vi "Heat Flow Front Panel.vi"(3 "Temp Control":dbl) -> (11 "Temp Indicator":dbl)   [LabVIEW 2019, in "Test Stands.lvlib" / "Heat Flow Test Stand.lvclass"]
uses:
  Heat Flow Test Stand.lvclass
panel:
  out "Heater dU":dbl format="%#.3f"
  out "Hot Side I":dbl format="%#.3f"
  out "I Res dU":dbl format="%#.1f"
  in  "ColdSideVolts":dbl min=0.0 max=8.0 step=0.01
  in  "HotSideVolts":dbl min=0.0 max=8.0 step=0.01
  out "Hot Side Power":dbl format="%9.2f"
  out "Hot Side Temp":dbl format="%#.2f"
  out "Cold Side Temp":dbl format="%#.2f"
  out "T 1":dbl
  out "T 2":dbl
  out "T 3":dbl
  out "T 4":dbl
  out "T 5":dbl
  out "T 6":dbl
  out "T 7":dbl
  out "T 8":dbl
  # "K"
  # "mV"
  # "A"
  # "V"
  # "K"
  # "W"
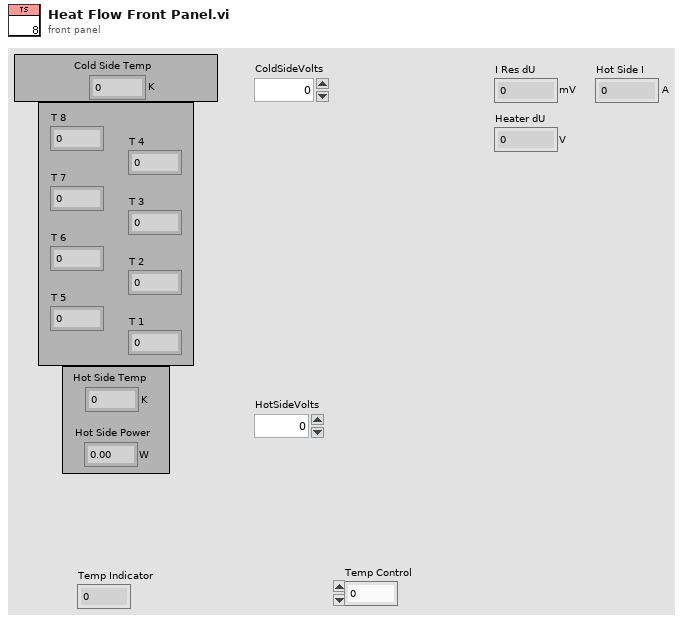
[diagram p1: front panel]
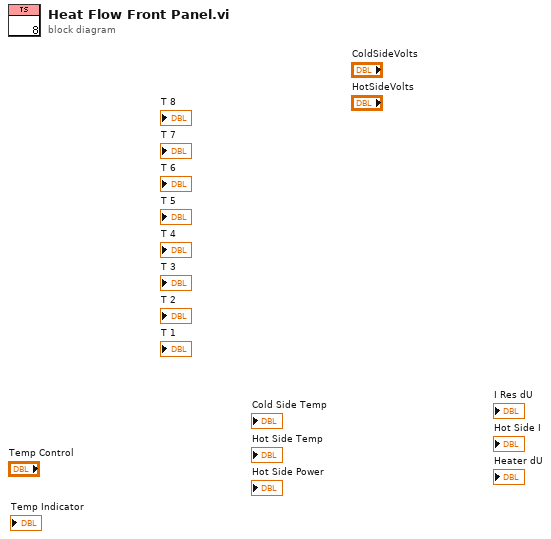
[diagram p0: block diagram]
diagram:
